vi "10.2.-Detección de Texto en Imágenes.vi"() -> ()   [LabVIEW 2020]
uses:
  <vilib>/Analysis/Matrix/Numeric/Conversions/Array To Matrix - RA2.vi
  <vilib>/Analysis/Matrix/Numeric/Multiply/Multiply - RM,RM.vi
  <vilib>/Analysis/Matrix/NI_Matrix.lvlib
panel:
  out "String":string
  in  "Path":path
  # "Visión Artificial - Detección de Texto en Imágenes\nDiego Cervantes Rodríguez\ndicer0.com"
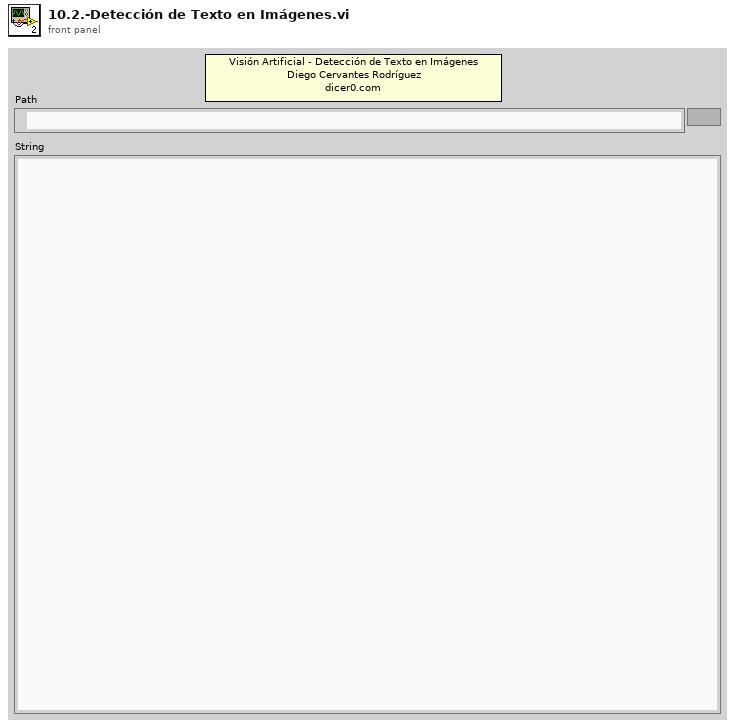
[diagram p1: front panel]
types:
  T1 = typedef "imagedata.ctl" = cluster{"image type":i32, "image depth":i32, "image":u8[], "mask":u8[], "colors":u32[], "Rectangle":cluster{"left":i16, "top":i16, "right":i16, "bottom":i16}}
  T2 = typedef "NI_Matrix.lvlib/RealMatrix.ctl" = dbl[][]
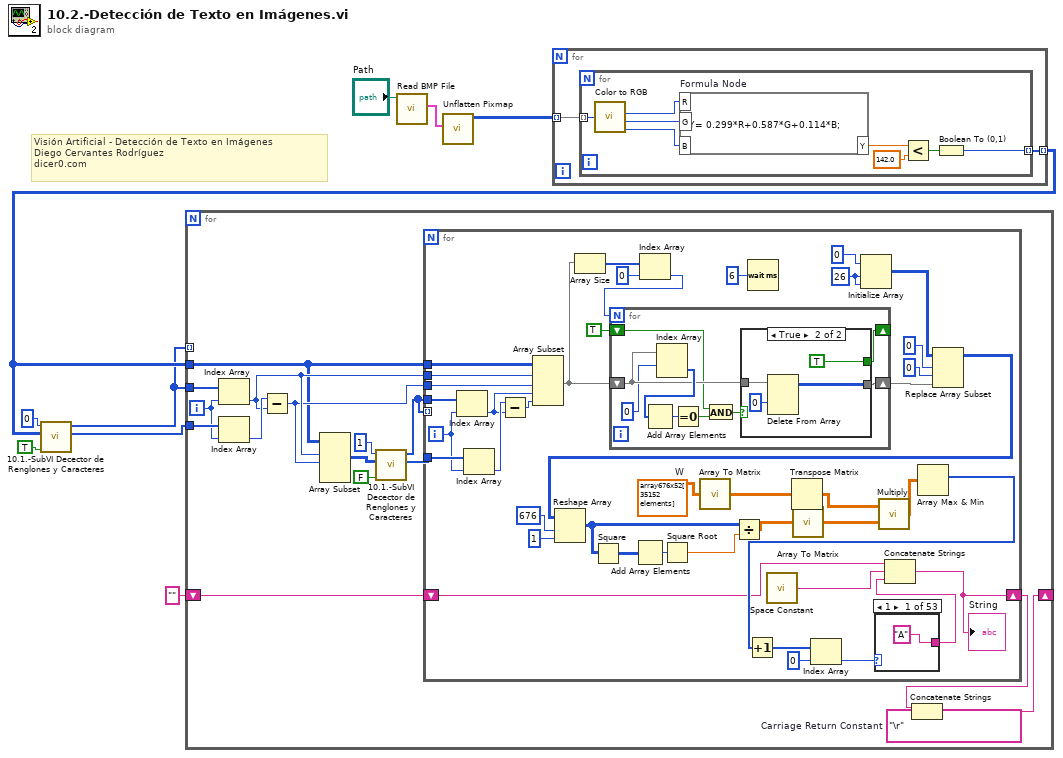
[diagram p0: block diagram]
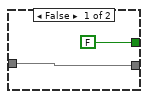
[diagram p2: hidden frame]
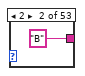
[diagram p3: hidden frame]
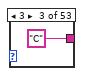
[diagram p4: hidden frame]
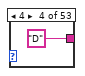
[diagram p5: hidden frame]
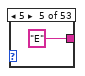
[diagram p6: hidden frame]
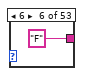
[diagram p7: hidden frame]
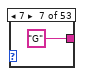
[diagram p8: hidden frame]
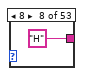
[diagram p9: hidden frame]
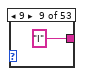
[diagram p10: hidden frame]
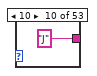
[diagram p11: hidden frame]
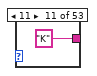
[diagram p12: hidden frame]
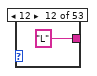
[diagram p13: hidden frame]
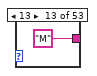
[diagram p14: hidden frame]
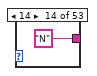
[diagram p15: hidden frame]
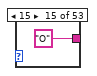
[diagram p16: hidden frame]
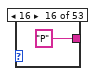
[diagram p17: hidden frame]
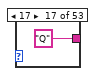
[diagram p18: hidden frame]
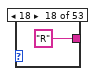
[diagram p19: hidden frame]
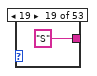
[diagram p20: hidden frame]
diagram:
  # "Visión Artificial - Detección de Texto en Imágenes\nDiego Cervantes Rodríguez\ndicer0.com"
  n1 = call <vilib>:"Read BMP File.vi"("path to BMP file"="Path") -> ("image data"=w9:T1)  [unwired: 8 in, 2 out]
  n2 = call <vilib>:"Unflatten Pixmap.vi"("image data"=w9) -> ("24-bit pixmap"=w8:u32[][])  [unwired: 4 in, 6 out]
  n3 = for {
    tunnel: w8 -> [w11] mode=indexing
    tunnel: [w10] -> w4 mode=indexing
    n4 = for {
      tunnel: w11 -> [w19] mode=indexing
      tunnel: [w12] -> w10 mode=indexing
      n5 = call <vilib>:"Color to RGB.vi"("Color"=w19) -> ("R"=w18:u8, "G"=w17:u8, "B"=w16:u8)  [unwired: 1 out]
      n6 = formula code="Y= 0.299*R+0.587*G+0.114*B;"("R"=w18, "G"=w17, "B"=w16) -> ("Y"=w15:dbl)
      n7 = Less?(x=w15, y=142.0) -> (x < y?=w13:bool)
      n8 = Boolean To (0,1)(Boolean=w13) -> (0, 1=w12:i16)
    }
  }
  n9 = call "10.1.-SubVI Decector de Renglones y Caracteres.vi"("Boolean"=TRUE, "ARREGLO"=w4, "INDICE"=0) -> ("FB"=w2:i32[], "FS"=w3:i32[])  [unwired: 7 in]
  n10 = for {
    tunnel: w2 -> [w35]
    tunnel: w3 -> [w34]
    tunnel: w4 -> [w21]
    shift-right: [w26] -> _
    shift-left: "" -> [w29]
    tunnel: w3 -> [_] mode=indexing
    i -> [w30]
    w27 = "\r"  # Carriage Return Constant
    n11 = Index Array(array=w34, index=w30) -> (element=w32:i32)
    n12 = Index Array(array=w35, index=w30) -> (element=w33:i32)
    n13 = Subtract(x=w33, y=w32) -> (x-y=w31:i32)
    n14 = Array Subset "Array Subset"(array=w21, index (row)=w32, length (row)=w31) -> (w24:i16[][])  [unwired: 2 in]
    n15 = call "10.1.-SubVI Decector de Renglones y Caracteres.vi"("Boolean"=FALSE, "ARREGLO"=w24, "INDICE"=1) -> ("FB"=w22:i32[], "FS"=w20:i32[])  [unwired: 7 in]
    n16 = for {
      tunnel: w21 -> [w77]
      tunnel: w32 -> [w76]
      tunnel: w31 -> [w75]
      tunnel: w20 -> [w73]
      tunnel: w22 -> [w72]
      shift-right: [w36] -> w28
      shift-left: w29 -> [w48]
      tunnel: w20 -> [_] mode=indexing
      i -> [w60]
      w37 = dbl[][] array676x52[35152 elements]  # W
      w69 = 26 ("dimension size")
      n17 = Index Array(array=w73, index=w60) -> (element=w71:i32)
      n18 = Index Array "Index Array"(array=w72, index=w60) -> (element=w74:i32)
      n19 = Subtract(x=w74, y=w71) -> (x-y=w70:i32)
      n20 = Array Subset "Array Subset"(array=w77, index (row)=w76, length (row)=w75, index (col)=w71, length (col)=w70) -> (w40:i16[][])
      n21 = Array Size(array=w40) -> (size(s)=w44:i32[])
      n22 = Index Array "Index Array"(array=w44, index=0) -> (element=w42:i32)
      n23 = for {
        N: w42 -> [_]
        shift-right: [w84] -> w39
        shift-left: w40 -> [w83]
        shift-right: [w81] -> _
        shift-left: TRUE -> [w79]
        n24 = Index Array "Index Array"(array=w83, index (row)=0) -> (element=w86:i16[])  [unwired: 1 in]
        n25 = Add Array Elements(numeric array=w86) -> (sum=w85:i16)
        n26 = Equal To 0?(x=w85) -> (x = 0?=w80:bool)
        n27 = And(x=w79, y=w80) -> (x .and. y?=w78:bool)
        n28 = case shown="True" w78 {
          tunnel: w83 -> [w88 w92]
          tunnel: [w88 w90] -> w84
          tunnel: [FALSE TRUE] -> w81
          frame False {
          }
          frame True {
            n29 = Delete From Array "Delete From Array"(array=w92, index (row)=0) -> (array with subset deleted=w90:i16[][])  [unwired: 2 in, 1 out]
          }
        }
      }
      n30 = call-poly <vilib>:"Array To Matrix.vi"("Real 2D Array"=w37) -> ("Real Matrix"=w59:T2)
      n31 = Wait (ms)(milliseconds to wait=u32 6) -> ()  [unwired: 1 out]
      n32 = call <vilib>:"Space Constant.vi"() -> ("String"=w49:string)
      n33 = Transpose Matrix(1:w59) -> (0:w56:T2)
      n34 = Initialize Array "Initialize Array"(u32 0 ("element"), w69, w69) -> (w53:u32[][])
      n35 = Replace Array Subset "Replace Array Subset"(array=w53, new element=w39, index (row)=0, index (col)=0 ("disabled index (col)")) -> (w45:u32[][])
      n36 = Reshape Array "Reshape Array"(w45, 676 ("dimension size"), 1 ("dimension size")) -> (w61:u32[][])
      n37 = Square(x=w61) -> (x^2=w64:u32[][])
      n38 = Add Array Elements(numeric array=w64) -> (sum=w63:u32)
      n39 = Square Root(x=w63) -> (sqrt(x)=w62:dbl)
      n40 = Divide(x=w61, y=w62) -> (x/y=w58:dbl[][])
      n41 = call-poly <vilib>:"Array To Matrix.vi"("Real 2D Array"=w58) -> ("Real Matrix"=w57:T2)
      n42 = call-poly <vilib>:"Multiply.vi"("Real Matrix B"=w57, "Real Matrix A"=w56) -> ("A * B"=w55:T2)
      n43 = Array Max & Min(array=w55) -> (max index (indices)=w54:i32[])  [unwired: 3 out]
      n44 = Increment(x=w54) -> (x+1=w51:i32[])
      n45 = Index Array "Index Array"(array=w51, index=0) -> (element=w46:i32)
      n46 = case shown="1" w46 {
        tunnel: ["A" "B" "C" "D" "E" "F" "G" "H" "I" "J" "K" "L" "M" "N" "O" "P" "Q" "R" "S" "T" "U" "V" "W" "X" "Y" "Z" "a" "b" "c" "d" "e" "f" "g" "h" "i" "j" "k" "l" "m" "n" "o" "p" "q" "r" "s" "t" "u" "v" "w" "x" "y" "z" w145] -> w47
        frame 1 {
        }
        frame 2 {
        }
        frame 3 {
        }
        frame 4 {
        }
        frame 5 {
        }
        frame 6 {
        }
        frame 7 {
        }
        frame 8 {
        }
        frame 9 {
        }
        frame 10 {
        }
        frame 11 {
        }
        frame 12 {
        }
        frame 13 {
        }
        frame 14 {
        }
        frame 15 {
        }
        frame 16 {
        }
        frame 17 {
        }
        frame 18 {
        }
        frame 19 {
        }
        frame 20 {
        }
        frame 21 {
        }
        frame 22 {
        }
        frame 23 {
        }
        frame 24 {
        }
        frame 25 {
        }
        frame 26 {
        }
        frame 27 {
        }
        frame 28 {
        }
        frame 29 {
        }
        frame 30 {
        }
        frame 31 {
        }
        frame 32 {
        }
        frame 33 {
        }
        frame 34 {
        }
        frame 35 {
        }
        frame 36 {
        }
        frame 37 {
        }
        frame 38 {
        }
        frame 39 {
        }
        frame 40 {
        }
        frame 41 {
        }
        frame 42 {
        }
        frame 43 {
        }
        frame 44 {
        }
        frame 45 {
        }
        frame 46 {
        }
        frame 47 {
        }
        frame 48 {
        }
        frame 49 {
        }
        frame 50 {
        }
        frame 51 {
        }
        frame 52 {
        }
        frame 0, Default {
          n47 = call <vilib>:"Space Constant.vi"() -> ("String"=w145:string)
        }
      }
      n48 = Concatenate Strings "Concatenate Strings"(w48, w49, w47) -> (w36:string)
      "String" <- w36
    }
    n49 = Concatenate Strings "Concatenate Strings"(w28, w27) -> (w26:string)
  }
